vi "Sort queue by Time to next scan.vi"(4 "Queue":T1(array[cluster]) {"Scan settings in queue" items=["Regular", "Inverted"]; "Time of the last scan (s)" format="%<%H:%M:%S>t"; "When did you stick it in?" format="%<%H:%M:%S>t"; "Time to next scan (s)" format="%<%H:%M:%S>t"; "Time in rig (s)" format="%<%H:%M:%S>t"}) -> (1 "Queue Out":T1(array[cluster]) {"Scan settings in queue" items=["Regular", "Inverted"]; "Time of the last scan (s)" format="%<%H:%M:%S>t"; "When did you stick it in?" format="%<%H:%M:%S>t"; "Time to next scan (s)" format="%<%H:%M:%S>t"; "Time in rig (s)" format="%<%H:%M:%S>t"})   [LabVIEW 2011]
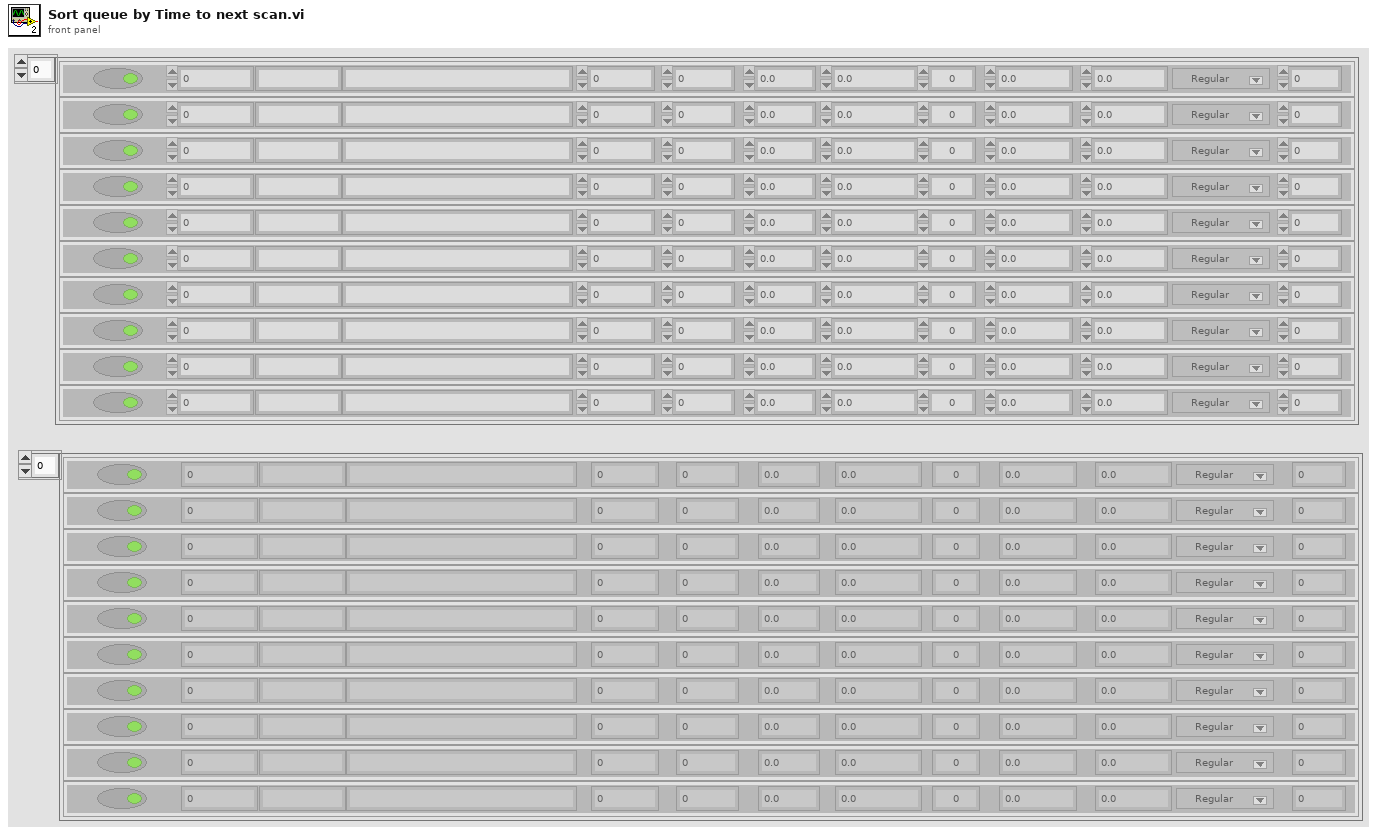
[diagram p1: front panel]
types:
  T1 = cluster{"Measure?":bool, "Area (cm^2)":dbl, "Cell Label":string, "Cell Description":string, "Cell Position":i32, "Time in rig (s)":dbl, "Time to next scan (s)":dbl, "Scan number":dbl, "When did you stick it in?":dbl, "Time between scans (s)":dbl, "Time of the last scan (s)":dbl, "Scan settings in queue":u16, "Sample Holder":dbl}[]
  T2 = cluster{"Time to next scan (s)":dbl, "Cluster":cluster{"Measure?":bool, "Area (cm^2)":dbl, "Cell Label":string, "Cell Description":string, "Cell Position":i32, "Time in rig (s)":dbl, "Time to next scan (s)":dbl, "Scan number":dbl, "When did you stick it in?":dbl, "Time between scans (s)":dbl, "Time of the last scan (s)":dbl, "Scan settings in queue":u16, "Sample Holder":dbl}}
  T3 = cluster{"Time to next scan (s)":dbl, "Cluster":cluster{"Measure?":bool, "Area (cm^2)":dbl, "Cell Label":string, "Cell Description":string, "Cell Position":i32, "Time in rig (s)":dbl, "Time to next scan (s)":dbl, "Scan number":dbl, "When did you stick it in?":dbl, "Time between scans (s)":dbl, "Time of the last scan (s)":dbl, "Scan settings in queue":u16, "Sample Holder":dbl}}[]
  T4 = cluster{"Measure?":bool, "Area (cm^2)":dbl, "Cell Label":string, "Cell Description":string, "Cell Position":i32, "Time in rig (s)":dbl, "Time to next scan (s)":dbl, "Scan number":dbl, "When did you stick it in?":dbl, "Time between scans (s)":dbl, "Time of the last scan (s)":dbl, "Scan settings in queue":u16, "Sample Holder":dbl}
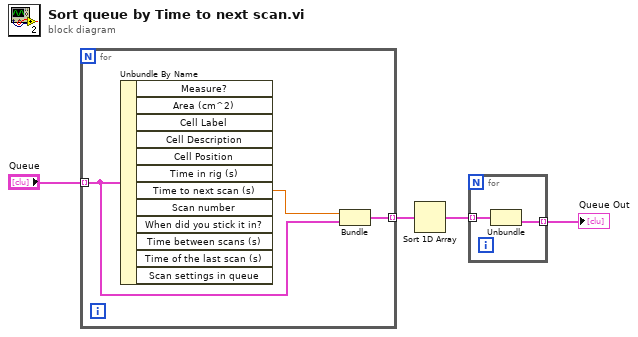
[diagram p0: block diagram]
diagram:
  n1 = for {
    tunnel: "Queue" -> [w6] mode=indexing
    tunnel: [w5] -> w4 mode=indexing
    n2 = Unbundle By Name(w6) -> ("Time to next scan (s)"=w7:dbl)  [unwired: 11 out]
    n3 = Bundle("Time to next scan (s)"=w7, "Cluster"=w6) -> (w5:T2)  [unwired: 1 in]
  }
  n4 = Sort 1D Array(array=w4) -> (sorted array=w3:T3)
  n5 = for {
    tunnel: w3 -> [w9] mode=indexing
    tunnel: [w8] -> w1 mode=indexing
    n6 = Unbundle(w9) -> ("Cluster"=w8:T4)  [unwired: 1 out]
  }
  "Queue Out" <- w1
